vi "BumpSetpoint.vi"(7 "Setpoint Name":string, 8 "Bump Down Trigger":bool, 9 "Bump Up Trigger":bool, 10 "Bump Increment":dbl, 11 "Original Setpoint":dbl) -> (2 "Bumped Setpoint":dbl)   [LabVIEW 2020]
doc: "Bumps a setpoint up or down by a specified interval"
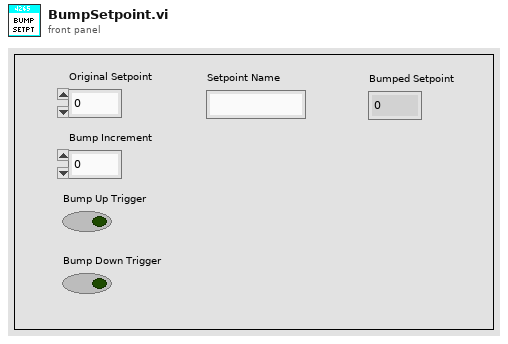
[diagram p1: front panel]
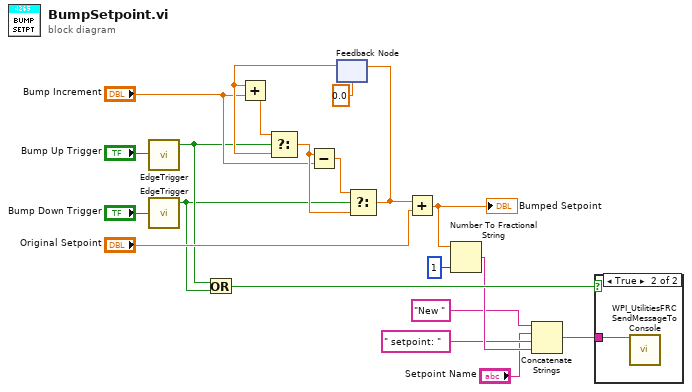
[diagram p0: block diagram]
diagram:
  n1 = call "EdgeTrigger.vi"("Input Signal"="Bump Up Trigger") -> ("Rising Edge Trigger"=w10:bool)  [unwired: 2 out]
  n2 = call "EdgeTrigger.vi"("Input Signal"="Bump Down Trigger") -> ("Rising Edge Trigger"=w9:bool)  [unwired: 2 out]
  n3 = Or(x=w10, y=w9) -> (x .or. y?=w8:bool)
  n4 = feedback #1(0.0) -> (w18:dbl)
  n5 = Add(x=w18, y="Bump Increment") -> (x+y=w15:dbl)
  n6 = Select(t=w15, s=w10, f=w18) -> (s? t:f=w19:dbl)
  n7 = Subtract(x=w19, y="Bump Increment") -> (x-y=w20:dbl)
  n8 = Select(t=w20, s=w9, f=w19) -> (s? t:f=w14:dbl)
  n9 = feedback-in #1(w14) -> ()
  n10 = Add(x=w14, y="Original Setpoint") -> (x+y=w7:dbl)
  "Bumped Setpoint" <- w7
  n11 = Number To Fractional String(number=w7, precision (6)=i16 1) -> (F-format string=w5:string)  [unwired: 2 in]
  n12 = Concatenate Strings("New " ("string"), "Setpoint Name", " setpoint: " ("string"), w5) -> (w2:string)
  n13 = case shown="True" w8 {
    tunnel: w2 -> [_ w21]
    frame False {
    }
    frame True {
      n14 = call <vilib>:"WPI_UtilitiesFRC SendMessageToConsole.vi"("Message"=w21) -> ()  [unwired: 14 in, 1 out]
    }
  }
